vi "Set and Wait to Restart Completion.vi"(8 "error in":errorcluster, 10 "IsRestarting Ref":refnum<vi>, 11 "Clear Ref":refnum<vi>) -> (0 "error out":errorcluster)   [LabVIEW 2025, in "Automotive Ethernet Bus Monitor UI.lvlib"]
doc: "Set IsRestart to True and trigger a Table Clear.\n\nThis VI not allows finishing completion till the IsRestart is False again (Restart was done)."
uses:
  Automotive Ethernet Bus Monitor UI.lvlib
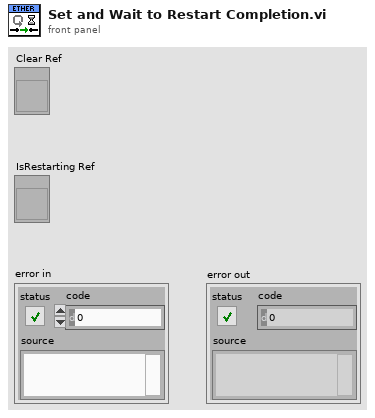
[diagram p1: front panel]
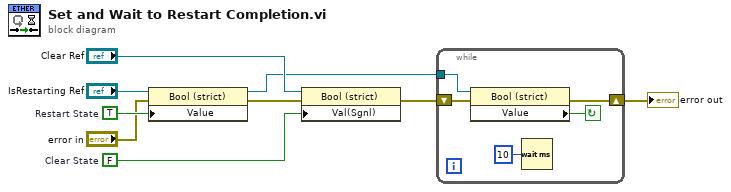
[diagram p0: block diagram]
diagram:
  w5 = FALSE  # Clear State
  w9 = TRUE  # Restart State
  n1 = property on="Property Node" class="Bool (strict)"(reference="IsRestarting Ref", error in="error in", "Value"=w9) -> (reference out=w3:refnum<vi>, error out=w8:errorcluster)
  n2 = property on="Property Node" class="Bool (strict)"(reference="Clear Ref", error in=w8, "Val(Sgnl)"=w5) -> (error out=w1:errorcluster)  [unwired: 1 out]
  n3 = while {
    tunnel: w3 -> [w14]
    shift-right: [w11] -> w2
    shift-left: w1 -> [w10]
    stop <- w13 continue-if-true
    n4 = property on="Property Node" class="Bool (strict)"(reference=w14, error in=w10) -> (error out=w11:errorcluster, "Value"=w13:bool)  [unwired: 1 out]
    n5 = Wait (ms)(milliseconds to wait=u32 10) -> ()  [unwired: 1 out]
  }
  "error out" <- w2
